vi "Impulse Decay Function.vi"(5 "Noise":dbl, 6 "Sigma":dbl, 7 "Offset":dbl, 8 "Tau":dbl, 9 "Amplitude":dbl, 10 "t0":dbl, 11 "NumSamp":u16=500) -> (3 "Array out":dbl[](array[numeric]))   [LabVIEW 2019, in "EmulatorActor.lvlib" / "EmulatorActor.lvclass"]
uses:
  EmulatorActor/EmulatorActor/EmulatorActor.lvclass
  <vilib>/gmath/NI_Gmath.lvlib
panel:
  out "Test Output":dbl[](graph)
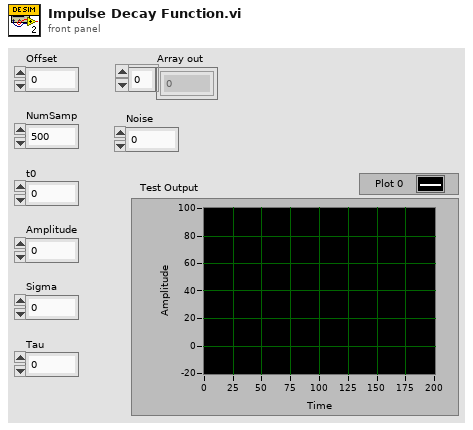
[diagram p1: front panel]
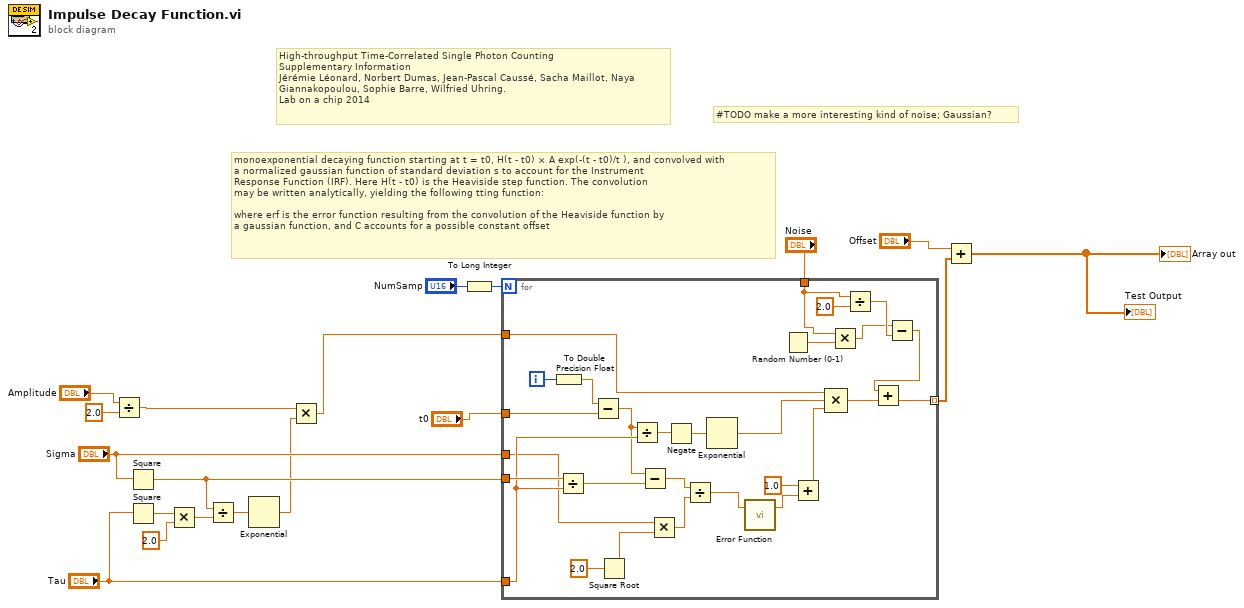
[diagram p0: block diagram]
diagram:
  # "#TODO make a more interesting kind of noise; Gaussian?"
  # "High-throughput Time-Correlated Single Photon Counting\nSupplementary Information\nJérémie Léonard, Norbert Dumas, Jean-Pascal Caussé, Sacha Maillot, Naya\nGiannakopoulou, Sophie Barre, Wilfried Uhring.\nLab on a chip 2014"
  # "monoexponential decaying function starting at t = t0, H(t - t0) × A exp(-(t - t0)/t ), and convolved with\na normalized gaussian function of standard deviation s to account for the Instrument\nResponse Function (IRF). Here H(t - t0) is the Heaviside step function. The convolution\nmay be written analytically, yielding the following tting function:\n\nwhere erf is the error function resulting from the convolution of the Heaviside function by\na gaussian function, and C accounts for a possible constant offset"
  n1 = Divide(x="Amplitude", y=2.0) -> (x/y=w7:dbl)
  n2 = Square(x="Sigma") -> (x^2=w16:dbl)
  n3 = Square(x="Tau") -> (x^2=w8:dbl)
  n4 = Multiply(x=w8, y=2.0) -> (x*y=w10:dbl)
  n5 = Divide(x=w16, y=w10) -> (x/y=w13:dbl)
  n6 = Exponential(1:w13) -> (0:w14:dbl)
  n7 = Multiply(x=w7, y=w14) -> (x*y=w15:dbl)
  n8 = To Long Integer(number="NumSamp") -> (32bit integer=w2:i32)
  n9 = for {
    N: w2 -> [_]
    tunnel: "t0" -> [w46]
    tunnel: "Tau" -> [w40]
    tunnel: w15 -> [w43]
    tunnel: w16 -> [w41]
    tunnel: "Sigma" -> [w33]
    tunnel: [w23] -> w18 mode=indexing
    tunnel: "Noise" -> [w21]
    i -> [w47]
    n10 = To Double Precision Float(number=w47) -> (double precision float=w20:dbl)
    n11 = Divide(x=w41, y=w40) -> (x/y=w38:dbl)
    n12 = Subtract(x=w20, y=w46) -> (x-y=w39:dbl)
    n13 = Square Root(x=2.0) -> (sqrt(x)=w34:dbl)
    n14 = Divide(x=w39, y=w40) -> (x/y=w45:dbl)
    n15 = Subtract(x=w39, y=w38) -> (x-y=w36:dbl)
    n16 = Multiply(x=w33, y=w34) -> (x*y=w32:dbl)
    n17 = Negate(x=w45) -> (-x=w44:dbl)
    n18 = Divide(x=w36, y=w32) -> (x/y=w37:dbl)
    n19 = Exponential(1:w44) -> (0:w42:dbl)
    n20 = call <vilib>:"Error Function.vi"("x"=w37) -> ("erf(x)"=w31:dbl)  [unwired: 2 in]
    n21 = Random Number (0-1)() -> (number: 0 to 1=w25:dbl)
    n22 = Add(x=1.0, y=w31) -> (x+y=w29:dbl)
    n23 = Compound Arithmetic op=MULTIPLY(w43, w42, w29) -> (w28:dbl)
    n24 = Multiply(x=w21, y=w25) -> (x*y=w26:dbl)
    n25 = Divide(x=w21, y=2.0) -> (x/y=w27:dbl)
    n26 = Subtract(x=w26, y=w27) -> (x-y=w22:dbl)
    n27 = Add(x=w22, y=w28) -> (x+y=w23:dbl)
  }
  n28 = Add(x="Offset", y=w18) -> (x+y=→"Array out" →"Test Output":dbl[])
